vi "test.vi"() -> ()   [LabVIEW 2012]
uses:
  <vilib>/Instr/_visa.llb/VISA Configure Serial Port (Instr).vi
panel:
  in  "Power":dbl
  out "Power":dbl
  out "Deg":dbl
  in  "Max_power":dbl
  in  "Min_power":dbl
  in  "Min_angle":dbl
  out "Numeric":i32
  out "Serial Settings:Number of Bytes at Serial Port":u32
  in  "Go":bool
  out "Position 2":i32
  in  "stop":bool
  out "Moving":bool
  out "Position":i32
  out "read buffer":string
  in  "baud rate":u32=9600
  in  "VISA resource name":refnum<visa-resource-name>="COM8"
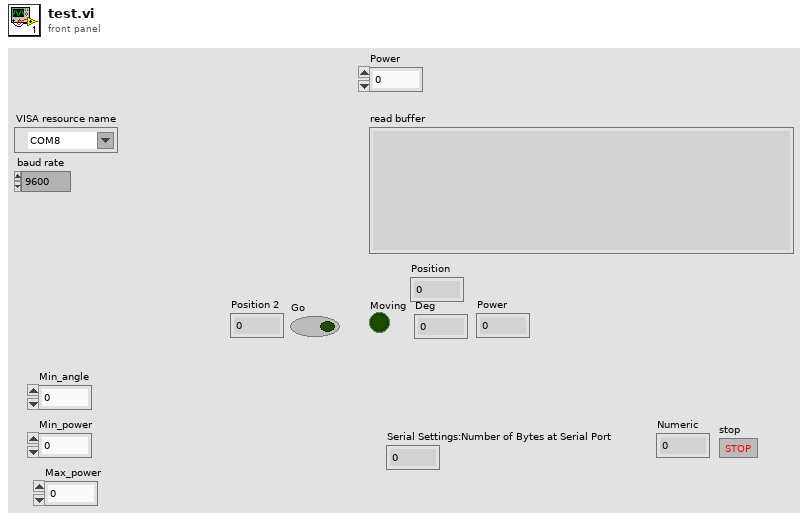
[diagram p1: front panel]
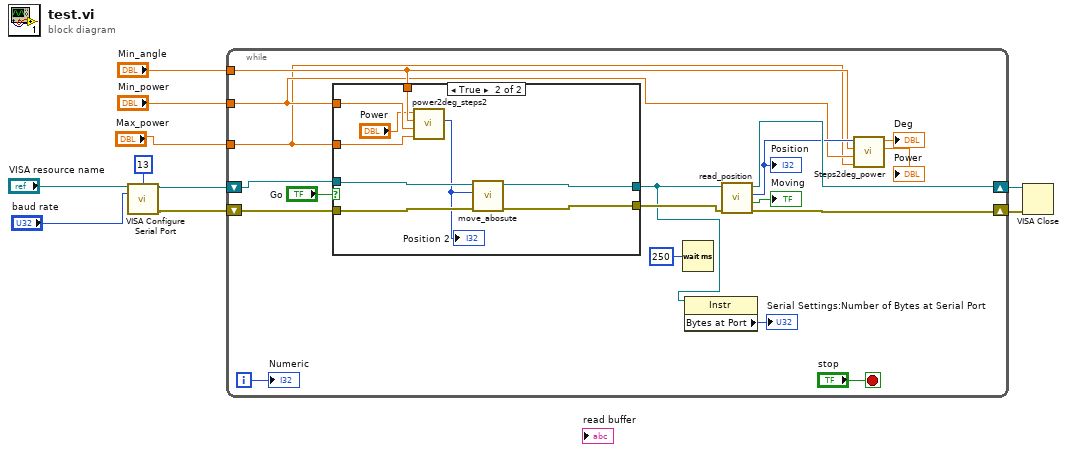
[diagram p0: block diagram]
diagram:
  n1 = call-poly "VISA Configure Serial Port"("VISA resource name"="VISA resource name", "termination char\n(0xA = '\\n' = LF)"=u8 13 ("termination char\n(0xA = '\\n' = LF)"), "baud rate (9600)"="baud rate") -> ("VISA resource name out"=w4:refnum<visa-resource-name>, "error out"=w5:errorcluster)  [unwired: 11 in]
  n2 = while {
    shift-right: [w28] -> w8
    shift-left: w4 -> [w23]
    shift-right: [w27] -> w7
    shift-left: w5 -> [w21]
    tunnel: "Min_angle" -> [w13]
    tunnel: "Min_power" -> [w12]
    tunnel: "Max_power" -> [w11]
    i -> [w17]
    stop <- "stop" stop-if-true
    n3 = case shown="True" "Go" {
      tunnel: w23 -> [w30 w39]
      tunnel: [w30 w38] -> w19
      tunnel: [w29 w37] -> w22
      tunnel: w21 -> [w29 w36]
      tunnel: w13 -> [_ w35]
      tunnel: w12 -> [_ w33]
      tunnel: w11 -> [_ w34]
      frame False {
      }
      frame True {
        n4 = call "power2deg_steps2.vi"("Max_power"=w34, "Min_power"=w33, "Min_angle"=w35, "Power"="Power") -> ("Steps"=w31:i32)  [unwired: 6 in, 1 out]
        "Position 2" <- w31
        n5 = call "move_abosute.vi"("error in (no error)"=w36, "Position"=w31, "VISA Refnum in"=w39) -> ("error out"=w37:errorcluster, "VISA Refnum out"=w38:refnum<visa-resource-name>)  [unwired: 7 in]
      }
    }
    n6 = Wait (ms)(milliseconds to wait=u32 250) -> ()  [unwired: 1 out]
    n7 = property class="Instr"(reference=w19) -> ("Bytes at Port"=→"Serial Settings:Number of Bytes at Serial Port":u32)  [unwired: 1 in, 2 out]
    n8 = call "read_position.vi"("error in (no error)"=w22, "VISA Refnum in"=w19) -> ("error out"=w27:errorcluster, "Moving"=→"Moving":bool, "Position"=w14:i32, "VISA Refnum out"=w28:refnum<visa-resource-name>)  [unwired: 6 in]
    "Position" <- w14
    n9 = call "Steps2deg_power.vi"("Max_power"=w11, "Min_power"=w12, "Min_angle"=w13, "Steps"=w14) -> ("Power"=→"Power":dbl, "Deg"=→"Deg":dbl)  [unwired: 6 in]
    "Numeric" <- w17
  }
  n10 = VISA Close(VISA resource name=w8, error in (no error)=w7) -> ()  [unwired: 1 out]
